vi "isSegmentCharacter.vi"(11 "characters":string) -> (3 "pchar":bool)   [LabVIEW 2013, in "openURI.lvlib"]
uses:
  openURI.lvlib
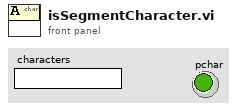
[diagram p1: front panel]
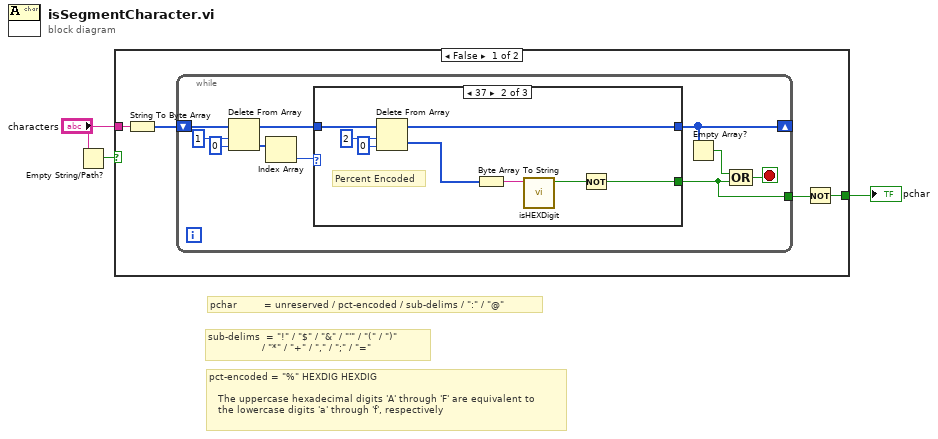
[diagram p0: block diagram]
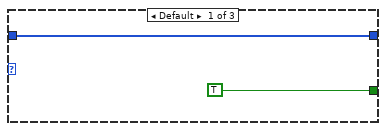
[diagram p2: hidden frame]
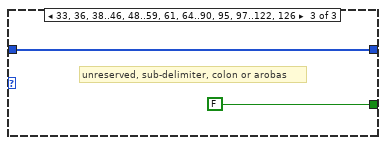
[diagram p3: hidden frame]
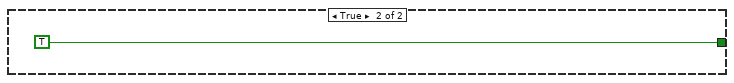
[diagram p4: hidden frame]
diagram:
  # "pct-encoded = \"%\" HEXDIG HEXDIG\n\n   The uppercase hexadecimal digits 'A' through 'F' are equivalent to\n   the lowercase digits 'a' through 'f', respectively"
  # "sub-delims  = \"!\" / \"$\" / \"&\" / \"'\" / \"(\" / \")\"\n                  / \"*\" / \"+\" / \",\" / \";\" / \"=\""
  # "pchar         = unreserved / pct-encoded / sub-delims / \":\" / \"@\""
  n1 = Empty String/Path?(string/path="characters") -> (empty?=w2:bool)
  n2 = case shown="False" w2 {
    tunnel: "characters" -> [w7 _]
    tunnel: [w4 TRUE] -> w3
    frame False {
      n3 = String To Byte Array(string=w7) -> (unsigned byte array=w6:u8[])
      n4 = while {
        shift-right: [w11] -> _
        shift-left: w6 -> [w17]
        tunnel: [w8] -> w5
        stop <- w9 stop-if-true
        n5 = Delete From Array(array=w17, length=1, index=0) -> (deleted portion=w14:u8[], array with subset deleted=w12:u8[])
        n6 = Index Array(array=w14) -> (element=w13:u8)  [unwired: 1 in]
        n7 = case shown="37" w13 {
          tunnel: w12 -> [w19 w25 w29]
          tunnel: [w19 w24 w29] -> w11
          tunnel: [TRUE w20 FALSE] -> w8
          frame Default {
          }
          frame 37 {
            # "Percent Encoded"
            n8 = Delete From Array(array=w25, length=2, index=0) -> (deleted portion=w23:u8[], array with subset deleted=w24:u8[])
            n9 = Byte Array To String(unsigned byte array=w23) -> (string=w22:string)
            n10 = call "isHEXDigit.vi"("characters"=w22) -> ("HEX Digits"=w21:bool)  [unwired: 10 in]
            n11 = Not(x=w21) -> (.not. x?=w20:bool)
          }
          frame 33, 36, 38..46, 48..59, 61, 64..90, 95, 97..122, 126 {
            # "unreserved, sub-delimiter, colon or arobas"
          }
        }
        n12 = Empty Array?(array=w11) -> (empty?=w10:bool)
        n13 = Compound Arithmetic op=OR(w10, w8) -> (w9:bool)
      }
      n14 = Not(x=w5) -> (.not. x?=w4:bool)
    }
    frame True {
    }
  }
  "pchar" <- w3
